vi "9linearconv.vi"() -> ()   [LabVIEW 2013]
uses:
  <vilib>/Analysis/2dsp.llb/1D Convolution (DBL).vi
  <vilib>/Analysis/NI_AALPro.lvlib
panel:
  out "Array 2":dbl[](array[numeric])
  out "Array":dbl[](array[numeric])
  out "Waveform Graph 3":dbl[](graph)
  out "Waveform Graph 2":dbl[](graph)
  out "Waveform Graph":dbl[](graph)
  in  "Y(n)":dbl[](array[numeric])
  in  "X(n)":dbl[](array[numeric])
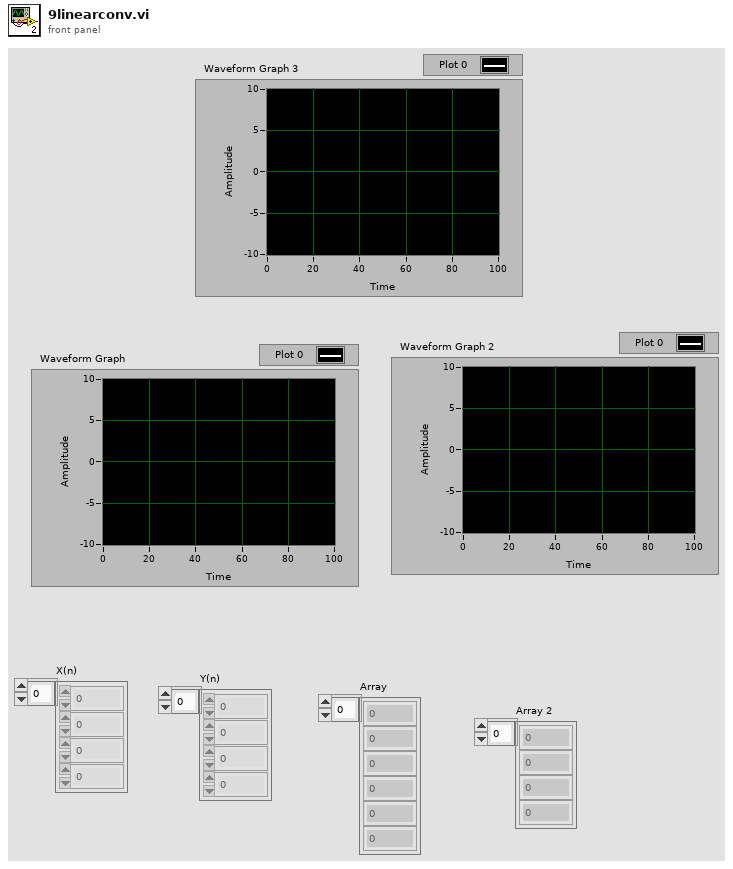
[diagram p1: front panel]
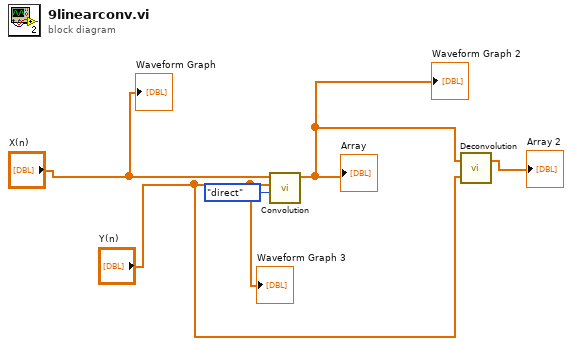
[diagram p0: block diagram]
diagram:
  n1 = call-poly <vilib>:"Convolution.vi"("algorithm"=enum32{"direct", "frequency domain"}."direct", "Y"="Y(n)", "X"="X(n)") -> ("X * Y"=w3:dbl[])  [unwired: 7 in, 1 out]
  "Waveform Graph 2" <- w3
  "Array" <- w3
  n2 = call <vilib>:"Deconvolution.vi"("Y"="Y(n)", "X * Y"=w3) -> ("X"=→"Array 2":dbl[])  [unwired: 1 out]
  "Waveform Graph" <- "X(n)"
  "Waveform Graph 3" <- "Y(n)"
